vi "Create.vi"(5 "Package in":refnum<class "Package.lvclass">, 8 "error in (no error)":errorcluster, 11 "Name":string) -> (0 "error out":errorcluster, 3 "Package":refnum<class "Package.lvclass">)   [LabVIEW 2017, in "Cobertura.lvlib" / "Package.lvclass"]
uses:
  Package.lvclass
  Package.lvclass/Package.ctl
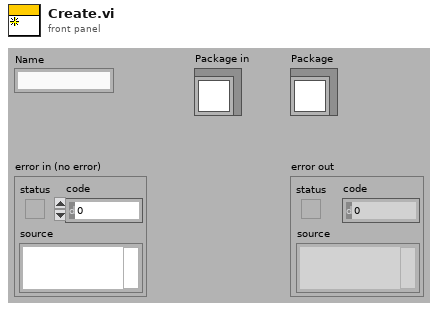
[diagram p1: front panel]
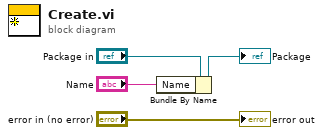
[diagram p0: block diagram]
diagram:
  n1 = Bundle By Name(cluster="Package in", "Name"="Name") -> (→"Package":refnum<class "Package.lvclass">)
  "error out" <- "error in (no error)"
